vi "get_data_exp.vi"(8 "error in (no error)":errorcluster, 11 "Experiment.lvclass in":refnum<class "Experiment.lvclass">) -> (0 "error out":errorcluster, 2 "Data":sgl[][](array[numeric]), 3 "Experiment.lvclass out":refnum<class "Experiment.lvclass">)   [LabVIEW 2019, in "Experiment.lvclass"]
uses:
  Experiment.lvclass
  Experiment.lvclass/Experiment.ctl
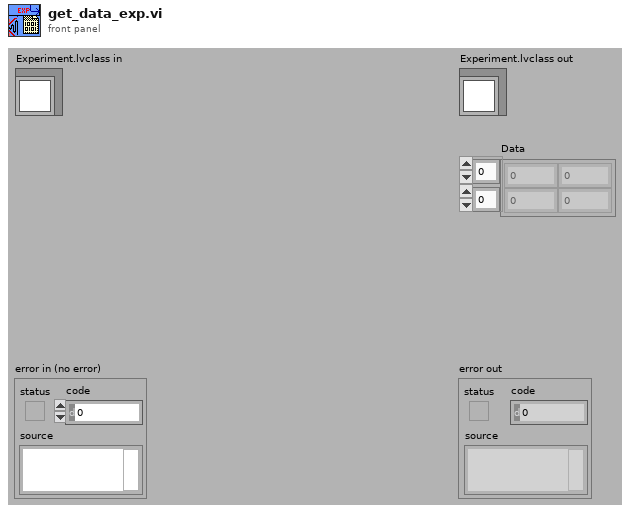
[diagram p1: front panel]
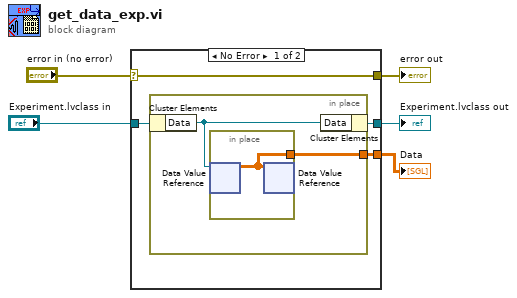
[diagram p0: block diagram]
diagram:
  n1 = case shown="No Error" "error in (no error)" {
    selector: "error in (no error)" -> [w9 w13]
    tunnel: [w9 w13] -> w4
    tunnel: [w6 w14] -> w2
    tunnel: "Experiment.lvclass in" -> [w8 w14]
    tunnel: [w7 _] -> w1
    frame No Error {
      n2 = in-place {
        in-place-border: [w11] -> w7
        n3 = in-place-cluster #1(w8) -> ("Data"=w10:refnum<data-value>)
        n4 = in-place {
          in-place-border: [w12] -> w11
          n5 = in-place-dvr #2(w10) -> (w12:sgl[][])  [unwired: 1 out]
          n6 = in-place-dvr #2(w12) -> ()  [unwired: 2 out]
        }
        n7 = in-place-cluster #1("Data"=w10) -> (w6:refnum<class "Experiment.lvclass">)
      }
    }
    frame Error {
    }
  }
  "error out" <- w4
  "Experiment.lvclass out" <- w2
  "Data" <- w1
